vi "AO Buffer Write (binary array).vi"(1 "channel state in (empty)":T1(array[ring]), 4 "buffer number\n(-1: no change)":i32=-1, 5 "time limit\n(-1: auto calculate)":sgl=-1.0 format="%0.2f", 6 "regeneration mode (0: no change)":u16(ring) items=["no change", "allow regeneration ", "do not allow regeneration", "stop after one generation"], 7 "alternate data and mode set (no change)":T3={"reserved"=[], "unused"=-1, "unused 1"=0, "write offset"=-1, "write mode"=enum."no change"}, 8 "error in (no error)":errorcluster, 9 "binary data (empty)":i16[][](array[numeric]), 10 "channel indices (empty)":u32[](array[numeric]), 11 "task ID":u32 format="%x") -> (0 "error out":errorcluster, 2 "update progress":T2={"buffer  number"=0, "output mark"=0, "write mark"=0, "buffer iterations"=0, "buffer  state"=enum."no such buffer", "channel state"=[enum."clear"]}, 3 "task ID out":u32 format="%x")   [LabVIEW 2009]
doc: "Writes analog <B>output</B> data to buffers created by the AO Buffer Config VI."
uses:
  <vilib>/Daq/lvdaq.dll
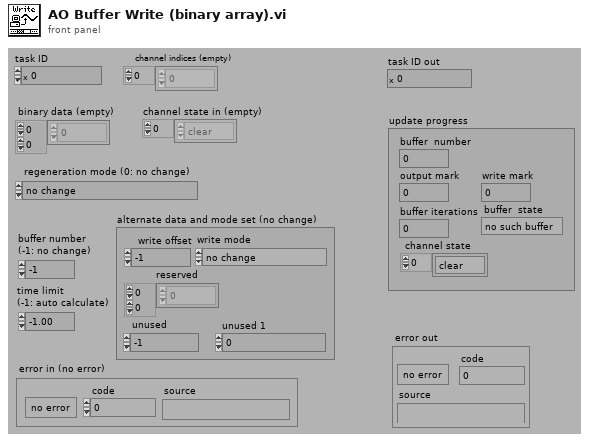
[diagram p1: front panel]
types:
  T1 = enum16{"clear", "running", "finished", "paused"}[]
  T2 = cluster{"buffer  number":i32, "output mark":i32, "write mark":i32, "buffer iterations":i32, "buffer  state":enum16{"no such buffer", "active", "finished", "waiting for data", "ready"}, "channel state":enum16{"clear", "running", "finished", "paused"}[]}
  T3 = cluster{"reserved":i16[][], "unused":i32, "unused 1":u32, "write offset":i32, "write mode":enum16{"no change", "relative to write mark", "relative to start of buffer"}}
  T4 = enum16{"no change", "relative to write mark", "relative to start of buffer"}
  T5 = cluster{i32, i32, i32, i32, u16, "channel state in (empty)":enum16{"clear", "running", "finished", "paused"}[]}
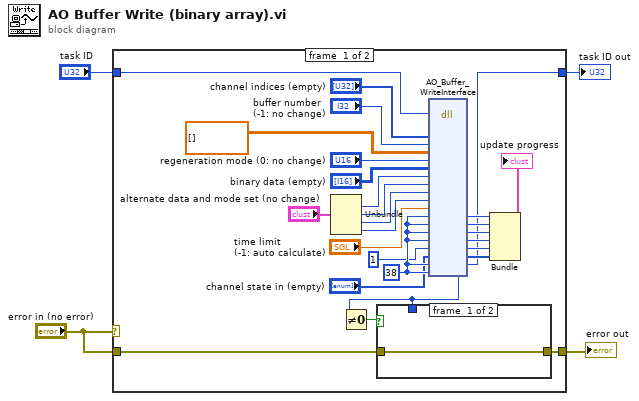
[diagram p0: block diagram]
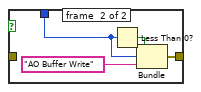
[diagram p2: hidden frame]
diagram:
  n1 = case shown="No Error" "error in (no error)" {
    tunnel: "task ID" -> [w14 w38]
    tunnel: [w13 w38] -> w3
    tunnel: [w9 w37] -> w2
    tunnel: "error in (no error)" -> [w8 w37]
    frame #0 {
      w31 = 38
      n2 = Unbundle("alternate data and mode set (no change)") -> ("unused"=w19:i32, "unused 1"=w20:u32, "write offset"=w21:i32, "write mode"=w22:T4)  [unwired: 1 out]
      n3 = dll-call lib="C:/Program Files/National Instruments/LabVIEW 2009/vi.lib/Daq/lvdaq.*" fn="AO_Buffer_WriteInterface"("task ID"=w14, "channel indices (empty)"="channel indices (empty)", "buffer number\n(-1: no change)"="buffer number\n(-1: no change)", "scaled data (empty)"=sgl[][] [], "regeneration mode (0: no change)"="regeneration mode (0: no change)", "binary data (empty)"="binary data (empty)", "unused"=w19, "unused 1"=w20, "write offset"=w21, "write mode"=w22, "time limit\n(-1: auto calculate)"="time limit\n(-1: auto calculate)", w31, w31, w31, w31, u16 1, "channel state in (empty)"="channel state in (empty)", w31, w31) -> (w26:i32, w27:i32, w28:i32, w25:i32, w24:u16, "channel state in (empty)"=w29:T1, w13:i32, w10:i32)  [unwired: 15 in, 2 out]
      n4 = Not Equal To 0?(x=w10) -> (x != 0?=w11:bool)
      n5 = case shown="True" w11 {
        tunnel: w10 -> [_ w34]
        tunnel: [w32 w33] -> w9
        tunnel: w8 -> [w32 _]
        frame #0 {
        }
        frame #1 {
          n6 = Less Than 0?(x=w34) -> (x < 0?=w36:bool)
          n7 = Bundle(w36, w34, "AO Buffer Write") -> (w33:errorcluster)  [unwired: 1 in]
        }
      }
      n8 = Bundle(w26, w27, w28, w25, w24, "channel state in (empty)"=w29) -> (→"update progress":T5)  [unwired: 1 in]
    }
    frame #1 {
    }
  }
  "task ID out" <- w3
  "error out" <- w2
